vi "Status Page.vi"(8 "Error In":errorcluster, 11 "Sample Test Template in":refnum<class "Sample Test Template.lvclass">) -> (0 "Error Out":errorcluster, 3 "Sample Test Template out":refnum<class "Sample Test Template.lvclass">)   [LabVIEW 2020, in "Sample Test Template.lvclass"]
doc: "Status page template"
uses:
  Sample Test Template.lvclass
  Typedef/User event controls.ctl
  Typedef/Queue Operation.ctl
  ADC DAC Test Measurement.lvlib
  INL DNL Test/INL DNL Test.lvclass
panel:
  # "Sample Status Page"
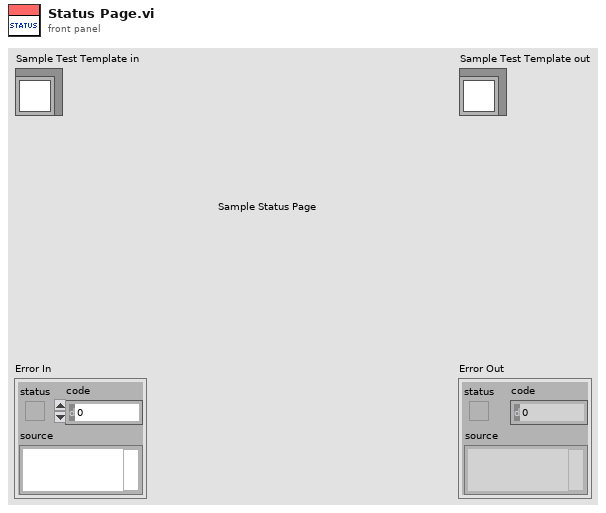
[diagram p1: front panel]
types:
  T1 = typedef "ADC DAC Test Measurement.lvlib/Queue Operation.ctl" = enum16{"Create Queue", "Enqueue", "Dequeue", "Enstack", "Flush Queue", "Release Queue"}
  T2 = typedef "ADC DAC Test Measurement.lvlib/User event controls.ctl" = enum16{"Create", "Generate", "Run Test", "Get Ref", "Destroy"}
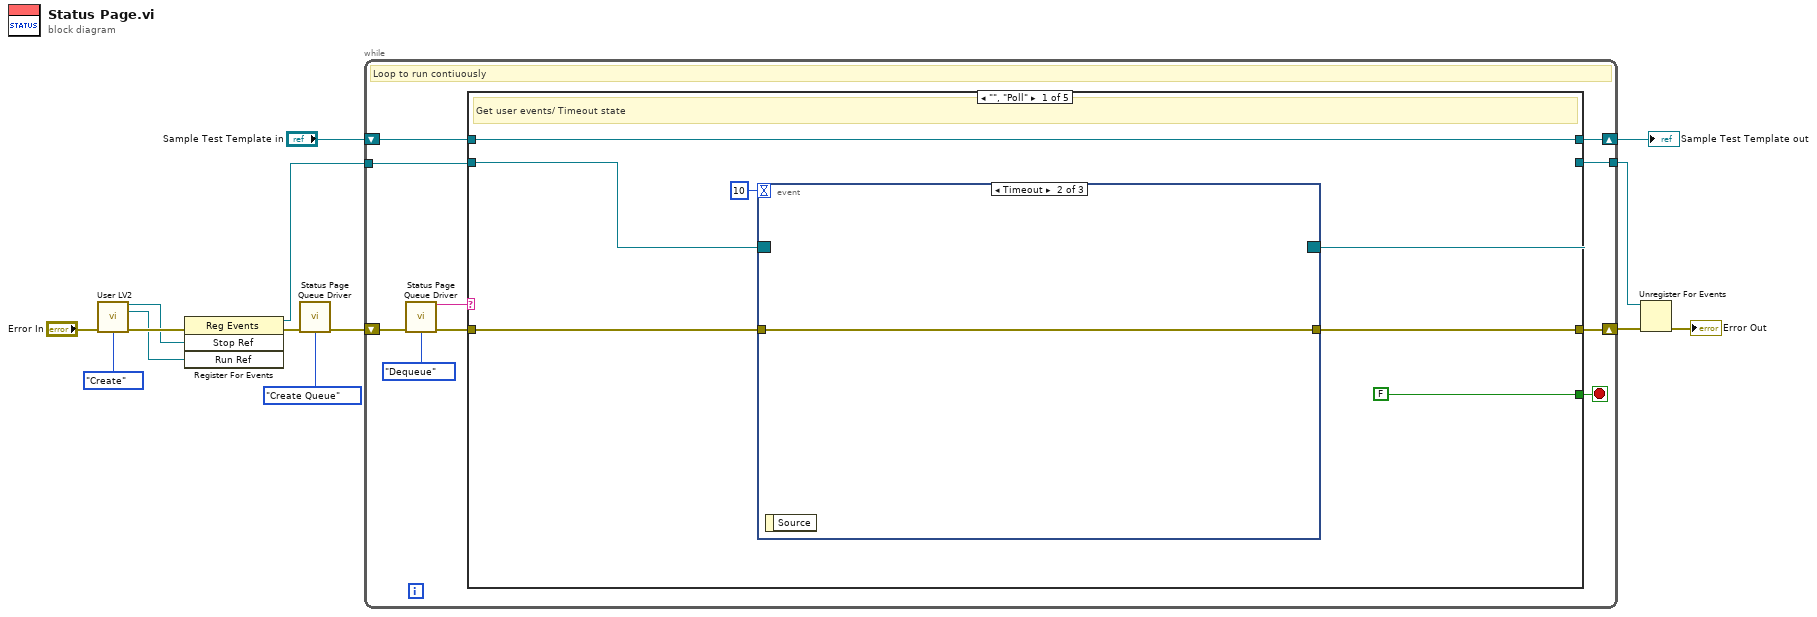
[diagram p0: block diagram]
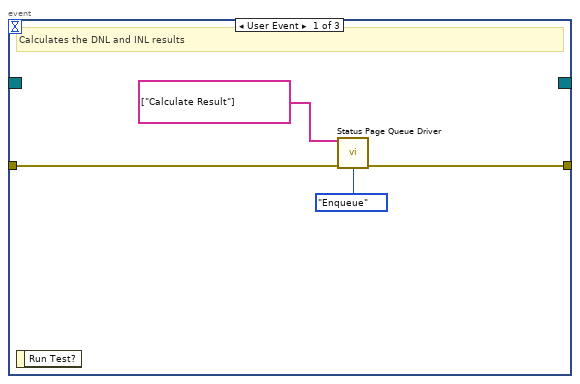
[diagram p2: hidden frame]
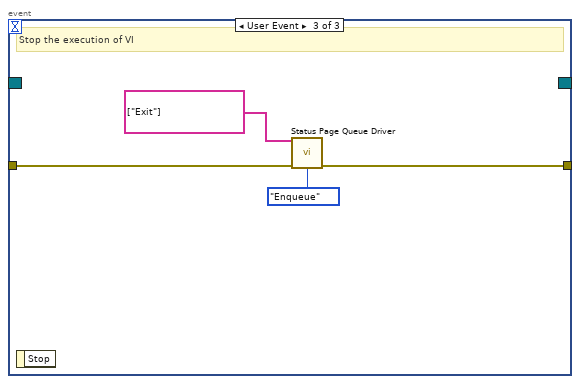
[diagram p3: hidden frame]
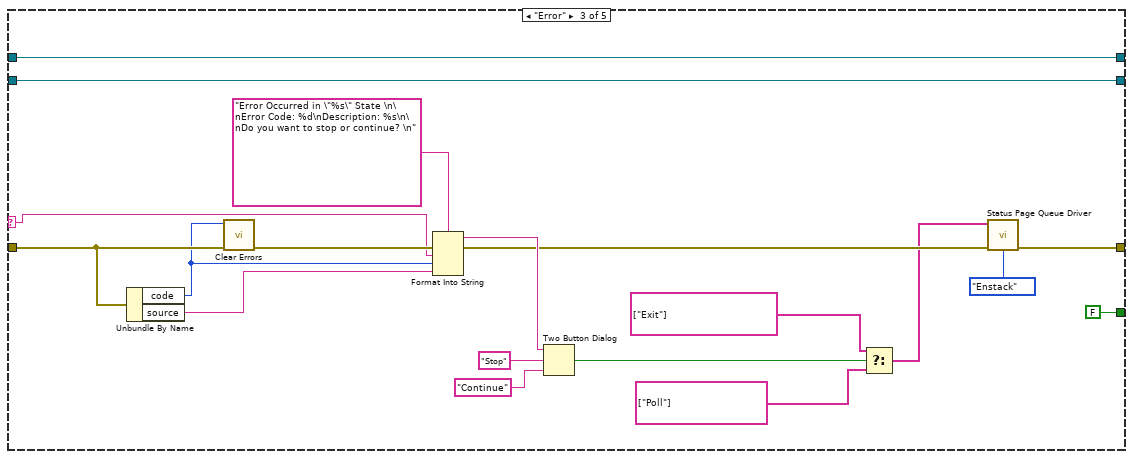
[diagram p5: hidden frame]
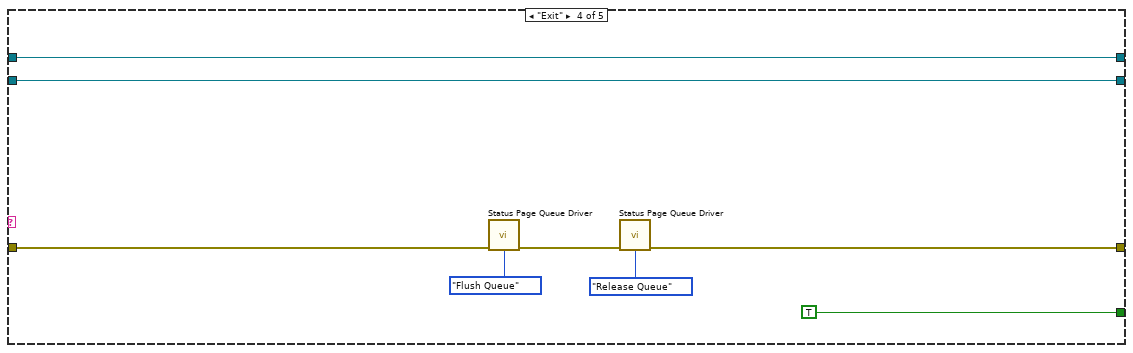
[diagram p6: hidden frame]
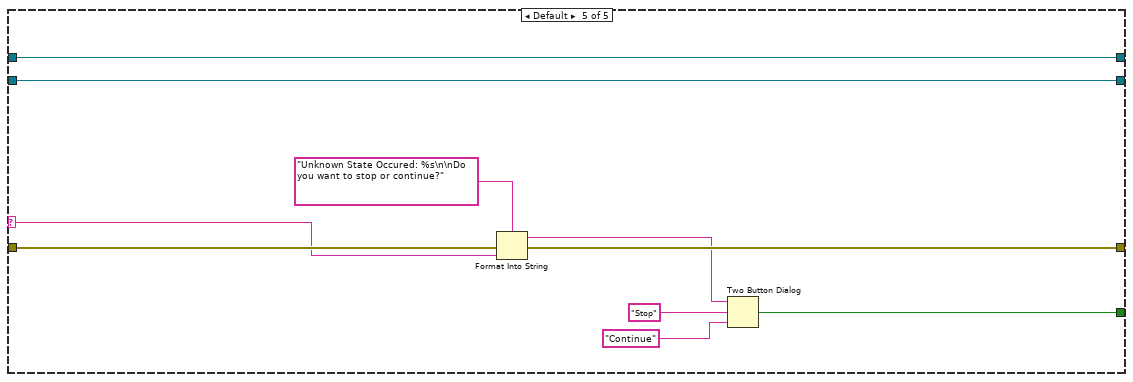
[diagram p7: hidden frame]
diagram:
  n1 = call "User LV2.vi"("Error In"="Error In", "User event controls"=User_event_controls."Create") -> ("Stop Ref"=w12:refnum<user-event>, "Run Ref"=w8:refnum<user-event>, "Error Out"=w13:errorcluster)  [unwired: 11 in]
  n2 = register-events(error in=w13, w12, w8) -> (reference out=w11:refnum<event-registration>, error out=w7:errorcluster)  [unwired: 1 in]
  n3 = call "Status Page Queue Driver.vi"("Error in"=w7, "Queue Operation"=Queue_Operation."Create Queue") -> ("Error out"=w5:errorcluster)  [unwired: 12 in, 1 out]
  n4 = while {
    shift-right: [w24] -> w10
    shift-left: w5 -> [w16]
    tunnel: w11 -> [w23]
    tunnel: [w21] -> w9
    shift-right: [w19] -> w3
    shift-left: "Sample Test Template in" -> [w20]
    stop <- w22 stop-if-true
    # "Loop to run contiuously"
    n5 = call "Status Page Queue Driver.vi"("Error in"=w16, "Queue Operation"=Queue_Operation."Dequeue") -> ("Dequeue Element"=w15:string, "Error out"=w17:errorcluster)  [unwired: 12 in]
    n6 = case shown="\"\", \"Poll\"" w15 {
      selector: w15 -> [_ _ w57 _ w75]
      tunnel: w17 -> [w31 w43 w59 w68 w80]
      tunnel: [w30 w43 w49 w64 w77] -> w24
      tunnel: w23 -> [w29 w42 w62 w70 w79]
      tunnel: [FALSE ("Stop") _ FALSE ("T button?") TRUE ("Stop") w71] -> w22
      tunnel: [w28 w42 w62 w70 w79] -> w21
      tunnel: w20 -> [w26 w41 w61 w69 w78]
      tunnel: [w26 w41 w61 w69 w78] -> w19
      frame "", "Poll" {
        # "Get user events/ Timeout state"
        n7 = event shown="[1] Timeout" {
          selector: w29 -> [_ _ _]
          dyn-events: [_ _ _] -> w28
          timeout: 10 -> [_ _ _]
          tunnel: w31 -> [w35 w36 w40]
          tunnel: [w34 w36 w39] -> w30
          event User Event {
            # "Calculates the DNL and INL results"
            n8 = event-data() -> ()  [unwired: 1 in, 1 out]
            n9 = call "Status Page Queue Driver.vi"("States"=string[] ["Calculate Result"], "Error in"=w35, "Queue Operation"=Queue_Operation."Enqueue") -> ("Error out"=w34:errorcluster)  [unwired: 11 in, 1 out]
          }
          event Timeout {
            n10 = event-data() -> ()  [unwired: 1 in, 1 out]
          }
          event User Event {
            # "Stop the execution of VI"
            n11 = event-data() -> ()  [unwired: 1 in, 1 out]
            n12 = call "Status Page Queue Driver.vi"("States"=string[] ["Exit"], "Error in"=w40, "Queue Operation"=Queue_Operation."Enqueue") -> ("Error out"=w39:errorcluster)  [unwired: 11 in, 1 out]
          }
        }
      }
      frame "Calculate Result" {
      }
      frame "Error" {
        n13 = Unbundle By Name(w59) -> ("code"=w56:i32, "source"=w55:string)
        n14 = call <vilib>:"Clear Errors.vi"("error in (no error)"=w59, "specific error code to clear (0: all)"=w56) -> ("error out"=w58:errorcluster)  [unwired: 4 in, 1 out]
        n15 = Format Into String(format string="Error Occurred in \"%s\" State \n\nError Code: %d\nDescription: %s\n\nDo you want to stop or continue? \n", error in=w58, w57, w56, w55) -> (resulting string=w54:string, error out=w50:errorcluster)  [unwired: 1 in]
        n16 = Two Button Dialog(message=w54, 1:"Continue" ("F button name (\"Cancel\")"), 2:"Stop" ("T button name (\"OK\")")) -> (T button?=w51:bool)
        n17 = Select(t=string[] ["Exit"] ("States"), s=w51, f=string[] ["Poll"]) -> (s? t:f=w46:string[])
        n18 = call "Status Page Queue Driver.vi"("States"=w46, "Error in"=w50, "Queue Operation"=Queue_Operation."Enstack") -> ("Error out"=w49:errorcluster)  [unwired: 11 in, 1 out]
      }
      frame "Exit" {
        n19 = call "Status Page Queue Driver.vi"("Error in"=w68, "Queue Operation"=Queue_Operation."Flush Queue") -> ("Error out"=w66:errorcluster)  [unwired: 12 in, 1 out]
        n20 = call "Status Page Queue Driver.vi"("Error in"=w66, "Queue Operation"=Queue_Operation."Release Queue") -> ("Error out"=w64:errorcluster)  [unwired: 12 in, 1 out]
      }
      frame Default {
        n21 = Format Into String(format string="Unknown State Occured: %s\n\nDo you want to stop or continue?", error in=w80, w75) -> (resulting string=w74:string, error out=w77:errorcluster)  [unwired: 1 in]
        n22 = Two Button Dialog(message=w74, 1:"Continue" ("F button name (\"Cancel\")"), 2:"Stop" ("T button name (\"OK\")")) -> (T button?=w71:bool)
      }
    }
  }
  "Sample Test Template out" <- w3
  n23 = Unregister For Events(event registration refnum=w9, error in=w10) -> (error out=→"Error Out":errorcluster)
